vi "Write Sample frequency.vi"(8 "error in (no error)":errorcluster, 10 "Sample frequency":dbl(knob)=8.0 scale=0.0..5.0, 11 "HRF_Device in":refnum<class "HRF_Device.lvclass">) -> (0 "error out":errorcluster, 3 "HRF_Device out":refnum<class "HRF_Device.lvclass">)   [LabVIEW 2020, in "HRF_Device.lvclass"]
uses:
  HRF_Device.lvclass
  HRF_Device.lvclass/HRF_Device.ctl
  D:/work/HackRF/Labview Driver/NetHackrf.dll
  NetHackrf.dll
  Read Device ref.vi
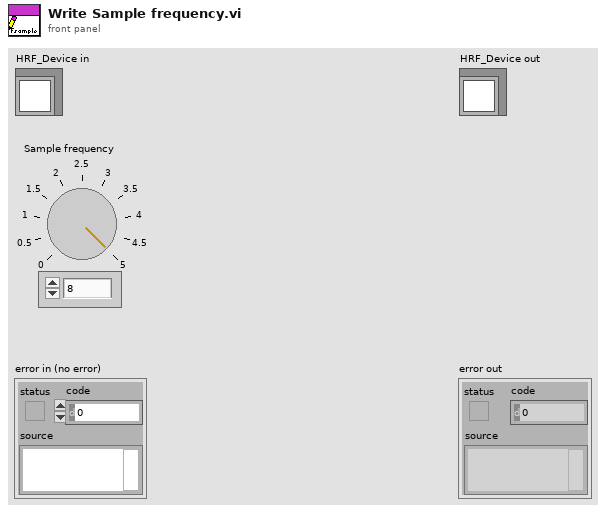
[diagram p1: front panel]
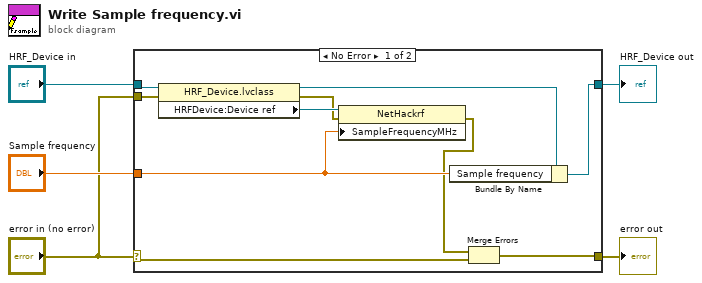
[diagram p0: block diagram]
diagram:
  n1 = case shown="No Error" "error in (no error)" {
    selector: "error in (no error)" -> [w8 w16]
    tunnel: [w6 w16] -> w5
    tunnel: [w15 w17] -> w3
    tunnel: "HRF_Device in" -> [w14 w17]
    tunnel: "Sample frequency" -> [w12 _]
    tunnel: "error in (no error)" -> [w9 _]
    frame No Error {
      n2 = property class="HRF_Device.lvclass"(reference=w14, error in=w9) -> (reference out=w13:refnum<class "HRF_Device.lvclass">, error out=w10:errorcluster, "HRFDevice:Device ref"=w11:refnum<k24>)
      n3 = property class="NetHackrf"(reference=w11, error in=w10, "SampleFrequencyMHz"=w12) -> (error out=w7:errorcluster)  [unwired: 1 out]
      n4 = Bundle By Name(cluster=w13, "Sample frequency"=w12) -> (w15:refnum<class "HRF_Device.lvclass">)
      n5 = Merge Errors(w7, w8) -> (w6:errorcluster)
    }
    frame Error {
    }
  }
  "error out" <- w5
  "HRF_Device out" <- w3
